vi "Report File Check.vi"(10 "Data Basic Path":path=path "S:/PNA_DATA/QSFP+  IBM 3m/Sample_#1_150331", 11 "File Name List":string[](array[string])=["SDD21", "SDD22", "SCD21"]) -> (3 "OK?":bool)   [LabVIEW 2011]
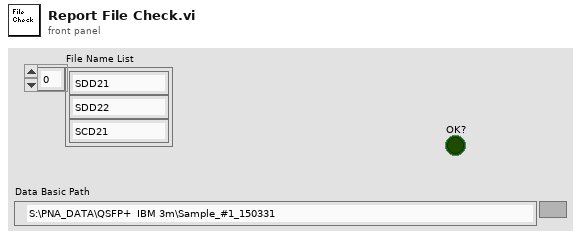
[diagram p1: front panel]
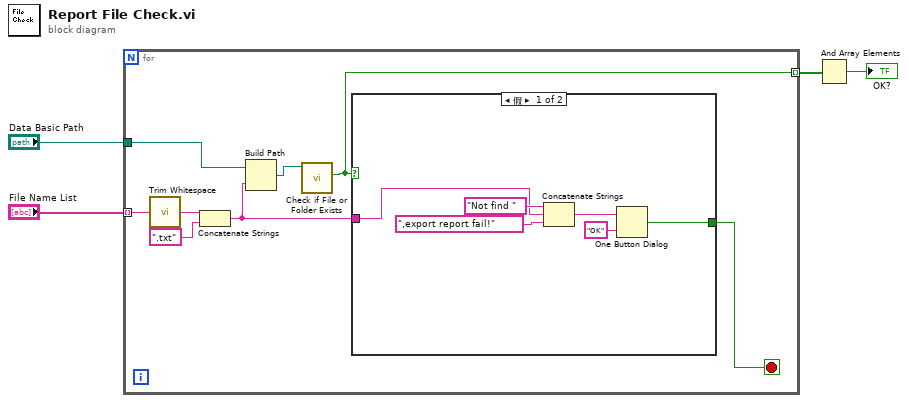
[diagram p0: block diagram]
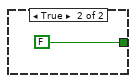
[diagram p2: hidden frame]
diagram:
  n1 = for {
    tunnel: "Data Basic Path" -> [w11]
    tunnel: "File Name List" -> [w6] mode=indexing
    tunnel: [w7] -> w2 mode=indexing
    stop <- w8 stop-if-true
    n2 = call <vilib>:"Trim Whitespace.vi"("string"=w6) -> ("trimmed string"=w5:string)  [unwired: 1 in]
    n3 = Concatenate Strings(w5, ".txt" ("字符串")) -> (w9:string)
    n4 = Build Path(base path=w11, name or relative path=w9) -> (appended path=w10:path)
    n5 = call <vilib>:"Check if File or Folder Exists.vi"("path"=w10) -> ("file or folder exists?"=w7:bool)  [unwired: 8 in, 2 out]
    n6 = case shown="假" w7 {
      tunnel: w9 -> [w16 _]
      tunnel: [w13 FALSE ("true")] -> w8
      frame False {
        n7 = Concatenate Strings("Not find " ("字符串"), w16, ",export report fail!" ("字符串")) -> (w14:string)
        n8 = One Button Dialog(message=w14, button name ("OK")="OK" ("按钮名称（“确定”）")) -> (true=w13:bool)
      }
      frame True {
      }
    }
  }
  n9 = And Array Elements(Boolean array=w2) -> (logical AND=→"OK?":bool)
